vi "SEK2020v1VI9PegarTubo.vi"(10 "NXT/EV3":T1) -> (2 "NXT/EV3 2":T1)   [LabVIEW 2016]
uses:
  <vilib>/NXT/Subs/LVHSConnector.ctl
  <vilib>/NXT/LegoClasses/BrickReference/BrickReference.lvclass
  <vilib>/NXT/Block Support/NXT_OutputPort.ctl
  <vilib>/NXT/NXTIO Xnodes/NXTIONodeSubVIs/NXTMoveMotors.vi
  <vilib>/NXT/NXTIO Xnodes/NXTIONodeSubVIs/NXTStopMotors.vi
  <vilib>/NXT/Dual Mode Library/Waits/Wait_Num.vi
  <vilib>/NXT/NXTIO Xnodes/AddressXNode/NXTIOAddress.xnode
  <vilib>/NXT/NXTIO Xnodes/NXTIOXNode/NXTIO.xnode
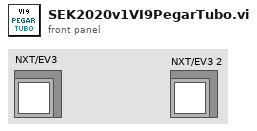
[diagram p1: front panel]
types:
  T1 = typedef "LVHSConnector.ctl" = refnum<class "BrickReference.lvclass">
  T2 = typedef "NXT_OutputPort.ctl" = u8
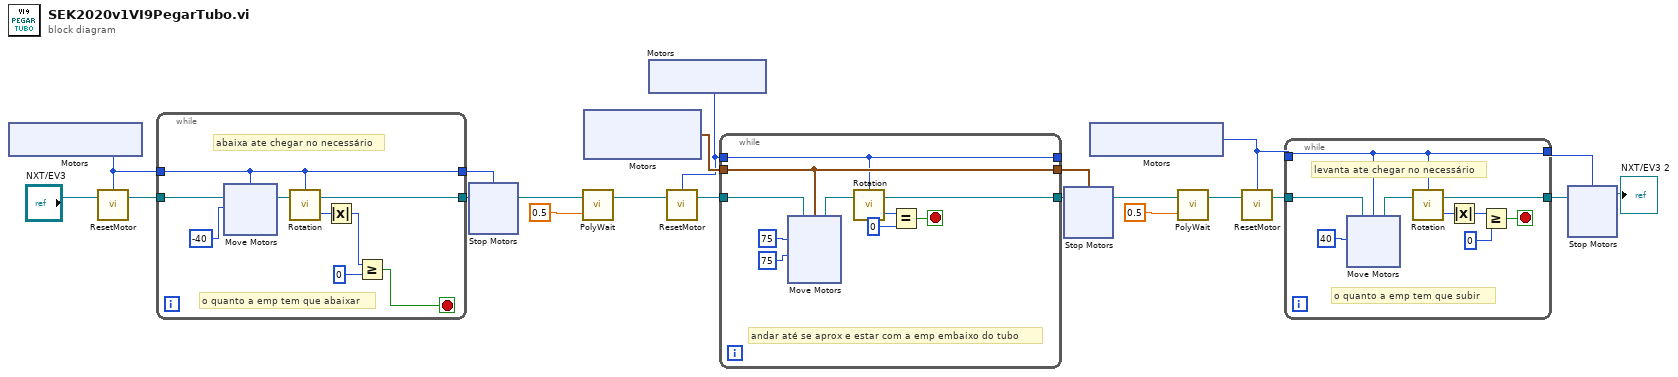
[diagram p0: block diagram]
diagram:
  n1 = xnode "Motors"() -> ("Motor"=w20:T2)
  n2 = call <vilib>:"ResetMotor.vi"("NXT/EV3"="NXT/EV3", "Port (All Ports)"=w20) -> ("NXT/EV3"=w21:T1)  [unwired: 2 in]
  n3 = while {
    tunnel: w21 -> [w30]
    tunnel: w20 -> [w28]
    tunnel: [w28] -> w19
    tunnel: [w26] -> w15
    stop <- w23 stop-if-true
    # "abaixa ate chegar no necessário"
    # "o quanto a emp tem que abaixar"
    n4 = xnode "Move Motors"("Power/Speed 1"=i8 -40, "Motors"=w28, "NXT/EV3"=w30) -> ("NXT/EV3"=w27:T1)
    n5 = call <vilib>:"Rotation.vi"("NXT/EV3"=w27, "Port (Port A)"=w28) -> ("Angle of Rotation"=w25:i32, "NXT/EV3"=w26:T1)  [unwired: 1 in]
    n6 = Absolute Value(x=w25) -> (abs(x)=w24:i32)
    n7 = Greater Or Equal?(x=w24, y=0) -> (x >= y?=w23:bool)
  }
  n8 = xnode "Stop Motors"("Motors"=w19, "NXT/EV3"=w15) -> ("NXT/EV3"=w7:T1)
  n9 = call-poly <vilib>:"PolyWait.vi"("Time (1 sec)"=sgl 0.5, "NXT/EV3"=w7) -> ("NXT/EV3"=w6:T1)  [unwired: 2 in]
  n10 = xnode "Motors"() -> ("Motor"=w18:cluster{"Port":T2, "Port":T2})
  n11 = xnode "Motors"() -> ("Motor"=w16:T2)
  n12 = call <vilib>:"ResetMotor.vi"("NXT/EV3"=w6, "Port (All Ports)"=w16) -> ("NXT/EV3"=w17:T1)  [unwired: 2 in]
  n13 = while {
    tunnel: w18 -> [w44]
    tunnel: [w40] -> w10
    tunnel: [w44] -> w9
    tunnel: w17 -> [w42]
    tunnel: w16 -> [w39]
    tunnel: [w39] -> _
    stop <- w46 stop-if-true
    # "andar até se aprox e estar com a emp embaixo do tubo"
    n14 = xnode "Move Motors"("Power/Speed 2"=i8 75, "Power/Speed 1"=i8 75, "Motors"=w44, "NXT/EV3"=w42) -> ("NXT/EV3"=w41:T1)
    n15 = call <vilib>:"Rotation.vi"("NXT/EV3"=w41, "Port (Port A)"=w39) -> ("Angle of Rotation"=w47:i32, "NXT/EV3"=w40:T1)  [unwired: 1 in]
    n16 = Equal?(x=w47, y=0) -> (x = y?=w46:bool)
  }
  n17 = xnode "Stop Motors"("Motors"=w9, "NXT/EV3"=w10) -> ("NXT/EV3"=w3:T1)
  n18 = xnode "Motors"() -> ("Motor"=w13:T2)
  n19 = call-poly <vilib>:"PolyWait.vi"("Time (1 sec)"=sgl 0.5, "NXT/EV3"=w3) -> ("NXT/EV3"=w4:T1)  [unwired: 2 in]
  n20 = call <vilib>:"ResetMotor.vi"("NXT/EV3"=w4, "Port (All Ports)"=w13) -> ("NXT/EV3"=w14:T1)  [unwired: 2 in]
  n21 = while {
    tunnel: w14 -> [w63]
    tunnel: w13 -> [w61]
    tunnel: [w61] -> w12
    tunnel: [w59] -> w11
    stop <- w64 stop-if-true
    # "o quanto a emp tem que subir"
    # "levanta ate chegar no necessário"
    n22 = xnode "Move Motors"("Power/Speed 1"=i8 40, "Motors"=w61, "NXT/EV3"=w63) -> ("NXT/EV3"=w60:T1)
    n23 = call <vilib>:"Rotation.vi"("NXT/EV3"=w60, "Port (Port A)"=w61) -> ("Angle of Rotation"=w58:i32, "NXT/EV3"=w59:T1)  [unwired: 1 in]
    n24 = Absolute Value(x=w58) -> (abs(x)=w57:i32)
    n25 = Greater Or Equal?(x=w57, y=0) -> (x >= y?=w64:bool)
  }
  n26 = xnode "Stop Motors"("Motors"=w12, "NXT/EV3"=w11) -> ("NXT/EV3"=→"NXT/EV3 2":T1)
